vi "Computer Name.vi"() -> (0 "Computer Name":string)   [LabVIEW 2014]
panel:
  # "LICENSED MATERIALS – PROPERTY OF IBM\nCopyright IBM Corp. 2016,\nALL RIGHTS RESERVED"
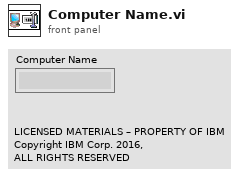
[diagram p1: front panel]
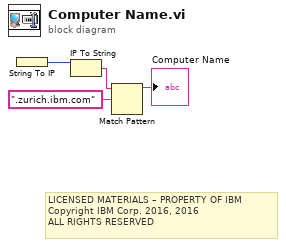
[diagram p0: block diagram]
diagram:
  # "LICENSED MATERIALS – PROPERTY OF IBM\nCopyright IBM Corp. 2016, 2016\nALL RIGHTS RESERVED"
  n1 = String To IP() -> (0:w4:u32)  [unwired: 1 in]
  n2 = IP To String(2:w4) -> (0:w3:string)  [unwired: 1 in]
  n3 = Match Pattern(string=w3, regular expression=".zurich.ibm.com") -> (before substring=→"Computer Name":string)  [unwired: 1 in, 3 out]
